vi "Listbox - In Progress.vi"(7 "Row to Update":i32, 8 "error in (no error)":errorcluster, 11 "SV B-M In":refnum<class "SV B-M (Host).lvclass">) -> (0 "error out":errorcluster, 3 "SV B-M Out":refnum<class "SV B-M (Host).lvclass">)   [LabVIEW 2015, in "SV B-M (Host).lvclass"]
doc: "Starts the timer in a test phase and updates the listbox for the active line to in progress."
uses:
  SV B-M (Host).lvclass
  SV B-M (Host).lvclass/SV B-M (Host).ctl
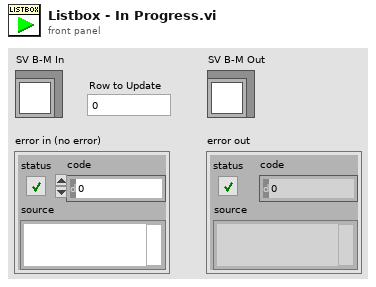
[diagram p1: front panel]
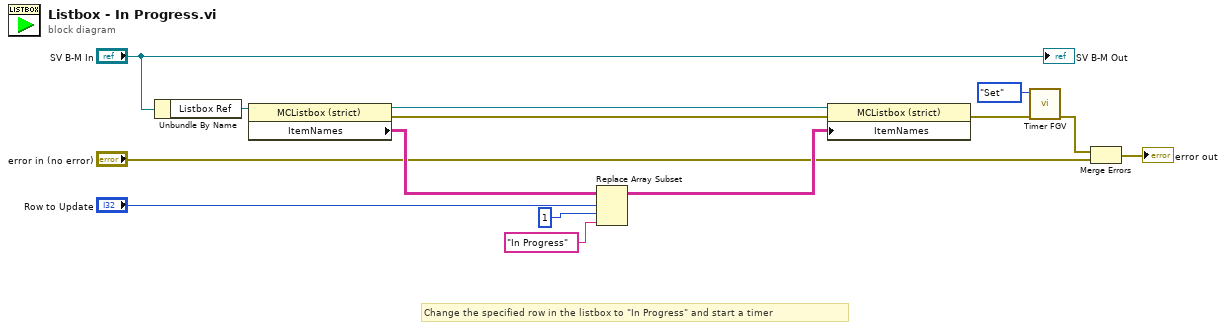
[diagram p0: block diagram]
diagram:
  # "Change the specified row in the listbox to \"In Progress\" and start a timer"
  n1 = Unbundle By Name("SV B-M In") -> ("Listbox Ref"=w12:refnum<vi>)
  n2 = property on="Property Node" class="MCListbox (strict)"(reference=w12) -> (reference out=w14:refnum<vi>, error out=w13:errorcluster, "ItemNames"=w6:string[][])  [unwired: 1 in]
  n3 = Replace Array Subset(array=w6, new element="In Progress", index (row)="Row to Update", index (col)=1 ("disabled index (col)")) -> (w5:string[][])
  n4 = property class="MCListbox (strict)"(reference=w14, error in=w13, "ItemNames"=w5) -> (error out=w9:errorcluster)  [unwired: 1 out]
  n5 = call "Timer FGV.vi"("error in (no error)"=w9, "Mode"=enum16{"Set", "Get"}."Set") -> ("error out"=w7:errorcluster)  [unwired: 8 in, 1 out]
  n6 = Merge Errors(w7, "error in (no error)") -> (→"error out":errorcluster)
  "SV B-M Out" <- "SV B-M In"
